vi "toJSON.vi"(8 "error in (no error)":errorcluster, 11 "tBSONBinary in":refnum<class "tBSONBinary.lvclass">) -> (0 "error out":errorcluster, 2 "JSON":string, 3 "tBSONBinary out":refnum<class "tBSONBinary.lvclass">)   [LabVIEW 2013, in "BSON.lvlib" / "tBSONBinary.lvclass"]
uses:
  tBSONBinary.lvclass
  tBSONElement/tBSONElement.lvclass
  getValue.vi
  BSON.lvlib
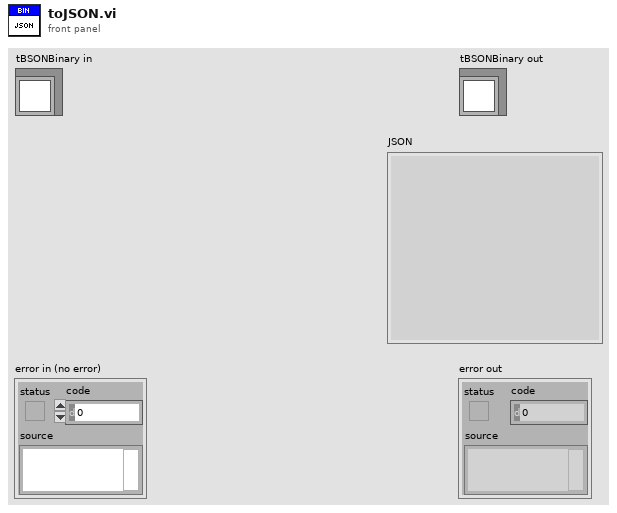
[diagram p1: front panel]
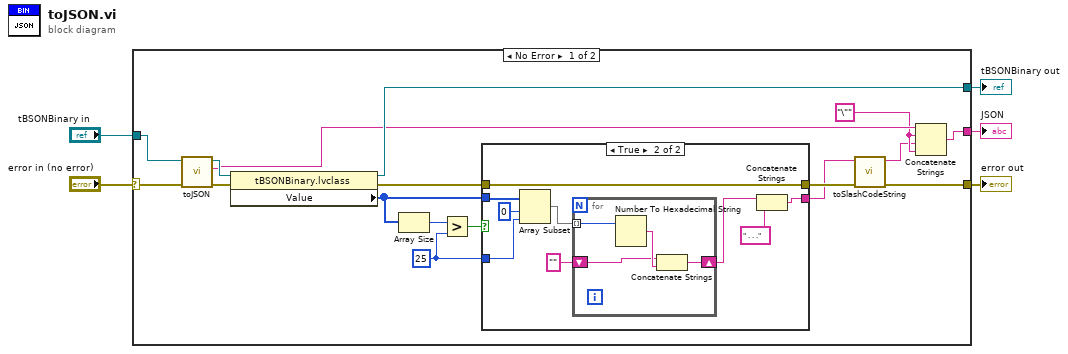
[diagram p0: block diagram]
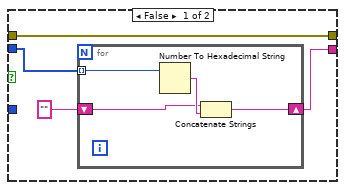
[diagram p2: hidden frame]
diagram:
  n1 = case shown="No Error" "error in (no error)" {
    selector: "error in (no error)" -> [w21 w44]
    tunnel: "tBSONBinary in" -> [w22 w45]
    tunnel: [w18 w45] -> w2
    tunnel: [w16 w44] -> w3
    tunnel: [w15 _] -> w1
    frame No Error {
      w7 = "\""
      w8 = 25 ("y")
      n2 = call-parent "toJSON.vi"("error in (no error)"=w21, "tBSONElement in"=w22) -> ("error out"=w20:errorcluster, "JSON"=w17:string, "tBSONElement out"=w19:refnum<class "tBSONBinary.lvclass">)  [unwired: 7 in]
      n3 = property class="tBSONBinary.lvclass"(reference=w19, error in=w20) -> (reference out=w18:refnum<class "tBSONBinary.lvclass">, error out=w11:errorcluster, "Value"=w12:u8[])
      n4 = Array Size(array=w12) -> (size(s)=w14:i32)
      n5 = Greater?(x=w14, y=w8) -> (0:w13:bool)
      n6 = case shown="True" w13 {
        tunnel: w12 -> [w25 w38]
        tunnel: w11 -> [w26 w39]
        tunnel: [w26 w39] -> w10
        tunnel: [w23 w35] -> w9
        tunnel: w8 -> [_ w36]
        frame False {
          n7 = for {
            tunnel: w25 -> [w30] mode=indexing
            shift-right: [w29] -> w23
            shift-left: "" -> [w27]
            n8 = Number To Hexadecimal String(2:w30) -> (0:w28:string)  [unwired: 1 in]
            n9 = Concatenate Strings(w27, w28) -> (w29:string)
          }
        }
        frame True {
          n10 = Array Subset(array=w38, index=0, length=w36) -> (w32:u8[])
          n11 = for {
            tunnel: w32 -> [w43] mode=indexing
            shift-right: [w42] -> w31
            shift-left: "" -> [w40]
            n12 = Number To Hexadecimal String(2:w43) -> (0:w41:string)  [unwired: 1 in]
            n13 = Concatenate Strings(w40, w41) -> (w42:string)
          }
          n14 = Concatenate Strings(w31, " . . ." ("string")) -> (w35:string)
        }
      }
      n15 = call "toSlashCodeString.vi"("error in (no error)"=w10, "String In"=w9) -> ("error out"=w16:errorcluster, "String Out"=w6:string)  [unwired: 8 in]
      n16 = Concatenate Strings(w17, w7, w6, w7) -> (w15:string)
    }
    frame Error {
    }
  }
  "error out" <- w3
  "tBSONBinary out" <- w2
  "JSON" <- w1
